vi "Test Assert Equal Type.vi"(8 "error in (no error)":errorcluster) -> (0 "error out":errorcluster)   [LabVIEW 2020]
uses:
  classes/Assert/Assert.lvclass
  classes/Test Suite/Test Suite.lvclass
  classes/Test/Test.lvclass
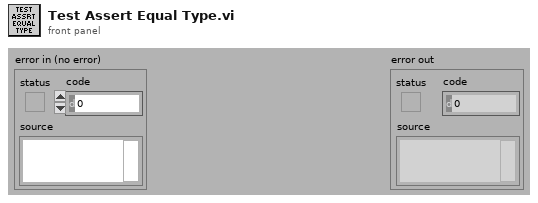
[diagram p1: front panel]
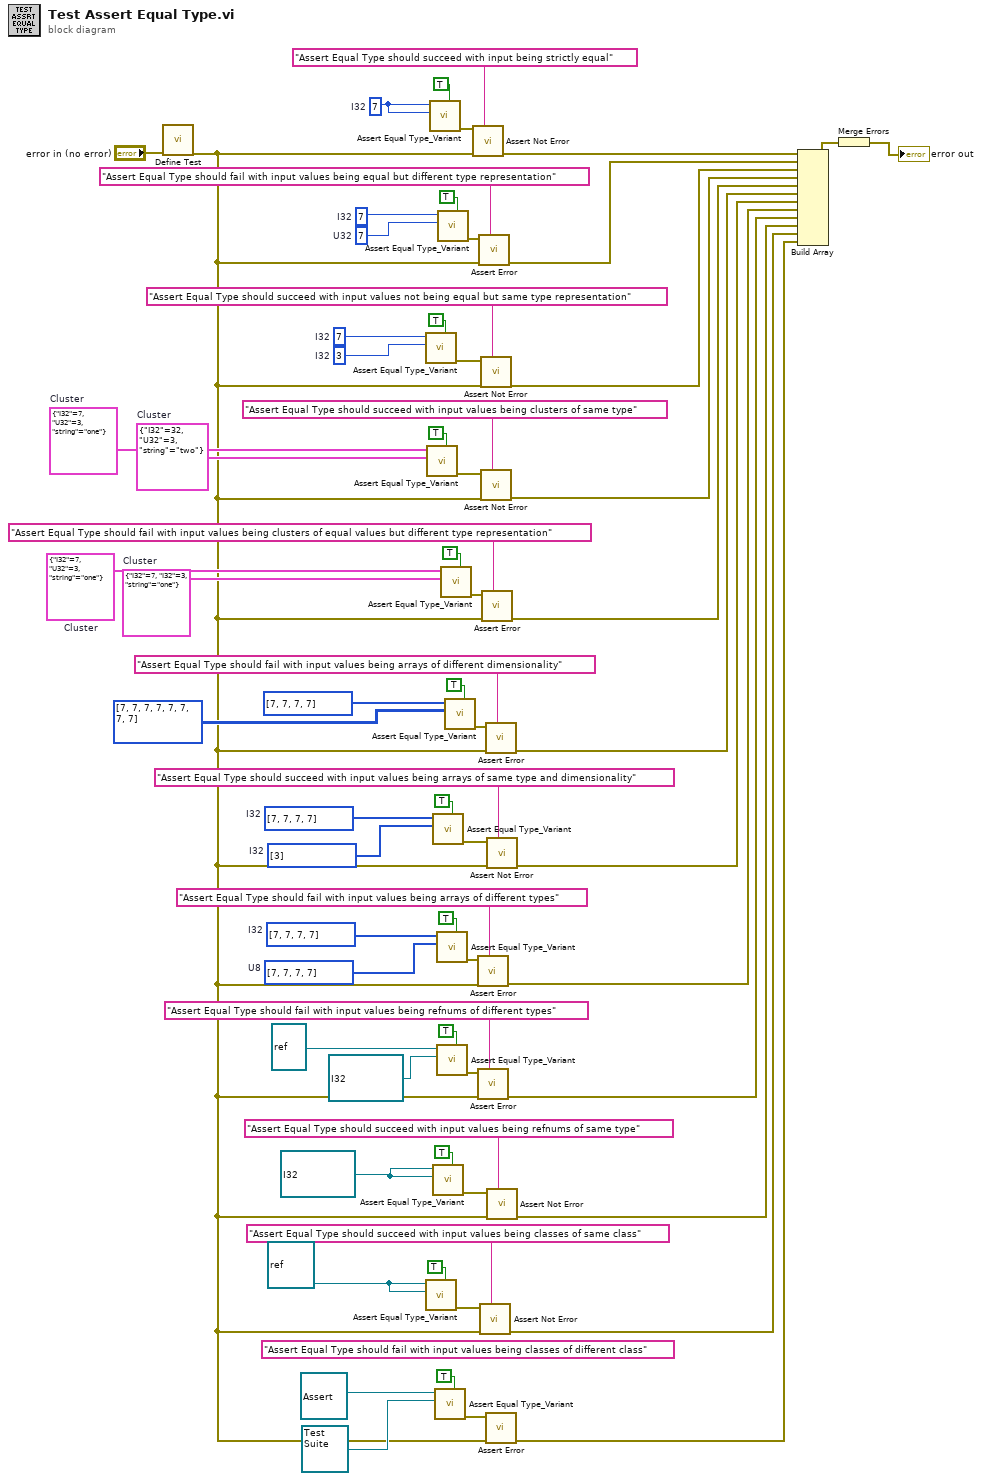
[diagram p0: block diagram]
diagram:
  (unwired) "Assert Equal Type should fail with input values being classes of different class" ("Label")
  w9 = refnum<class> refnum ("LabVIEW Object")
  w13 = refnum<queue> refnum ("queue out")
  w24 = u8[] [7, 7, 7, 7]  # U8
  w25 = i32[] [7, 7, 7, 7]  # I32
  w30 = i32[] [3]  # I32
  w31 = i32[] [7, 7, 7, 7]  # I32
  w50 = cluster{"I32":i32, "I32":i32, "string":string} {"I32"=7, "I32"=3, "string"="one"}  # Cluster
  w51 = cluster{"I32":i32, "U32":u32, "string":string} {"I32"=7, "U32"=3, "string"="one"}  # Cluster
  w43 = cluster{"I32":i32, "U32":u32, "string":string} {"I32"=32, "U32"=3, "string"="two"}  # Cluster
  w44 = cluster{"I32":i32, "U32":u32, "string":string} {"I32"=7, "U32"=3, "string"="one"}  # Cluster
  w59 = u32 7  # U32
  w60 = 7  # I32
  w63 = 7  # I32
  w47 = 3  # I32
  w48 = 7  # I32
  n1 = call "Define Test.vi"("error in (no error)"="error in (no error)") -> ("error out"=w2:errorcluster)  [unwired: 9 in, 1 out]
  n2 = call "Assert Equal Type_Variant.vi"("Assert Only? (F)"=TRUE, "Y"=w47, "X"=w48) -> ("error out"=w45:errorcluster)  [unwired: 7 in, 1 out]
  n3 = call "Assert Equal Type_Variant.vi"("Assert Only? (F)"=TRUE, "Y"=w9, "X"=w9) -> ("error out"=w10:errorcluster)  [unwired: 7 in, 1 out]
  n4 = call "Assert Equal Type_Variant.vi"("Assert Only? (F)"=TRUE, "Y"=w43, "X"=w44) -> ("error out"=w42:errorcluster)  [unwired: 7 in, 1 out]
  n5 = call "Assert Equal Type_Variant.vi"("Assert Only? (F)"=TRUE, "Y"=w63, "X"=w63) -> ("error out"=w61:errorcluster)  [unwired: 7 in, 1 out]
  n6 = call "Assert Equal Type_Variant.vi"("Assert Only? (F)"=TRUE, "Y"=w30, "X"=w31) -> ("error out"=w33:errorcluster)  [unwired: 7 in, 1 out]
  n7 = call "Assert Equal Type_Variant.vi"("Assert Only? (F)"=TRUE, "Y"=w13, "X"=w13) -> ("error out"=w15:errorcluster)  [unwired: 7 in, 1 out]
  n8 = call "Assert Equal Type_Variant.vi"("Assert Only? (F)"=TRUE, "Y"=refnum<class "Test Suite.lvclass"> refnum ("Caraya.lvlib:Test Suite.lvclass"), "X"=refnum<class "Assert.lvclass"> refnum ("Caraya.lvlib:Assert.lvclass")) -> ("error out"=w5:errorcluster)  [unwired: 7 in, 1 out]
  n9 = call "Assert Equal Type_Variant.vi"("Assert Only? (F)"=TRUE, "Y"=w24, "X"=w25) -> ("error out"=w28:errorcluster)  [unwired: 7 in, 1 out]
  n10 = call "Assert Equal Type_Variant.vi"("Assert Only? (F)"=TRUE, "Y"=refnum<queue> refnum ("queue out"), "X"=refnum<vi> refnum ("This VI")) -> ("error out"=w20:errorcluster)  [unwired: 7 in, 1 out]
  n11 = call "Assert Equal Type_Variant.vi"("Assert Only? (F)"=TRUE, "Y"=w59, "X"=w60) -> ("error out"=w57:errorcluster)  [unwired: 7 in, 1 out]
  n12 = call "Assert Equal Type_Variant.vi"("Assert Only? (F)"=TRUE, "Y"=w50, "X"=w51) -> ("error out"=w54:errorcluster)  [unwired: 7 in, 1 out]
  n13 = call "Assert Equal Type_Variant.vi"("Assert Only? (F)"=TRUE, "Y"=i32[][] [[7, 7, 7, 7], [7, 7, 7, 7]], "X"=i32[] [7, 7, 7, 7]) -> ("error out"=w38:errorcluster)  [unwired: 7 in, 1 out]
  n14 = call "Assert Not Error.vi"("Label"="Assert Equal Type should succeed with input being strictly equal", "error in (no error)"=w2, "Not Error?"=w61) -> ("error out"=w68:errorcluster)  [unwired: 7 in, 1 out]
  n15 = call "Assert Error.vi"("Label"="Assert Equal Type should fail with input values being arrays of different types", "error in (no error)"=w2, "Error?"=w28) -> ("error out"=w23:errorcluster)  [unwired: 7 in, 1 out]
  n16 = call "Assert Error.vi"("Label"="Assert Equal Type should fail with input values being refnums of different types", "error in (no error)"=w2, "Error?"=w20) -> ("error out"=w17:errorcluster)  [unwired: 7 in, 1 out]
  n17 = call "Assert Error.vi"("Label"="Assert Equal Type should fail with input values being equal but different type representation", "error in (no error)"=w2, "Error?"=w57) -> ("error out"=w67:errorcluster)  [unwired: 7 in, 1 out]
  n18 = call "Assert Not Error.vi"("Label"="Assert Equal Type should succeed with input values being classes of same class", "error in (no error)"=w2, "Not Error?"=w10) -> ("error out"=w7:errorcluster)  [unwired: 7 in, 1 out]
  n19 = call "Assert Not Error.vi"("Label"="Assert Equal Type should succeed with input values not being equal but same type representation", "error in (no error)"=w2, "Not Error?"=w45) -> ("error out"=w65:errorcluster)  [unwired: 7 in, 1 out]
  n20 = call "Assert Not Error.vi"("Label"="Assert Equal Type should succeed with input values being clusters of same type", "error in (no error)"=w2, "Not Error?"=w42) -> ("error out"=w55:errorcluster)  [unwired: 7 in, 1 out]
  n21 = call "Assert Error.vi"("Label"="Assert Equal Type should fail with input values being clusters of equal values but different type representation", "error in (no error)"=w2, "Error?"=w54) -> ("error out"=w49:errorcluster)  [unwired: 7 in, 1 out]
  n22 = call "Assert Error.vi"("Label"="Assert Equal Type should fail with input values being arrays of different dimensionality", "error in (no error)"=w2, "Error?"=w38) -> ("error out"=w37:errorcluster)  [unwired: 7 in, 1 out]
  n23 = call "Assert Error.vi"("error in (no error)"=w2, "Error?"=w5) -> ("error out"=w1:errorcluster)  [unwired: 8 in, 1 out]
  n24 = call "Assert Not Error.vi"("Label"="Assert Equal Type should succeed with input values being arrays of same type and dimensionality", "error in (no error)"=w2, "Not Error?"=w33) -> ("error out"=w29:errorcluster)  [unwired: 7 in, 1 out]
  n25 = call "Assert Not Error.vi"("Label"="Assert Equal Type should succeed with input values being refnums of same type", "error in (no error)"=w2, "Not Error?"=w15) -> ("error out"=w12:errorcluster)  [unwired: 7 in, 1 out]
  n26 = Build Array(w68, w67, w65, w55, w49, w37, w29, w23, w17, w12, w7, w1) -> (w66:errorcluster[])
  n27 = Merge Errors(w66) -> (→"error out":errorcluster)
